vi "CameraSetParams.vi"(8 "error in (no error)":errorcluster, 10 "settings":T2={"exposure"=0.0, "external"=FALSE, "roi"={"left"=0, "top"=0, "right"=0, "bottom"=0}, "frames"=0, "binning"={"x"=1, "y"=1}}, 11 "NIvision in":refnum<class "IMAQdx.lvclass">) -> (0 "error out":errorcluster, 1 "roi_out":T1, 2 "attributes":variant[](array[variant]), 3 "NIvision out":refnum<class "IMAQdx.lvclass">)   [LabVIEW 2010, in "IMAQdx.lvclass"]
uses:
  <userlib>/bias/classes/IMAQdx/IMAQdx.lvclass
  <userlib>/bias/subvis/ExposureSettings.ctl
  <userlib>/bias/subvis/ROI_rect.ctl
  <vilib>/vision/driver/IMAQdx.llb/IMAQdx Acquisition Mode.ctl
  <userlib>/bias/classes/IMAQdx/IMAQdx.lvclass/IMAQdx.ctl
  <vilib>/vision/driver/NI_Vision_Acquisition_Software.lvlib
  resource/objmgr/imaqdx.rc
panel:
  out "ValueDBL":dbl
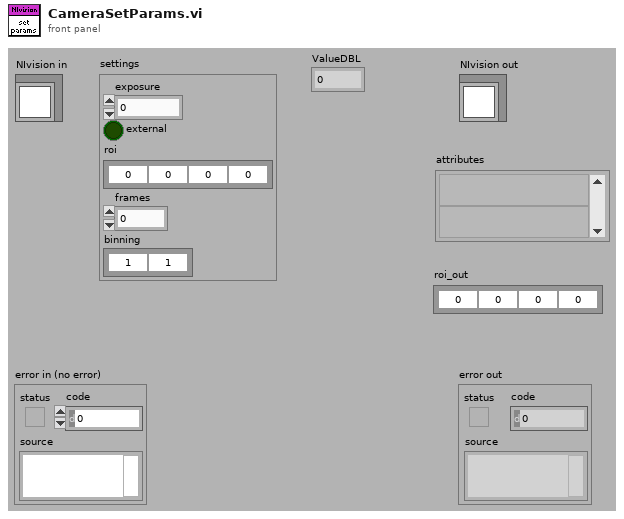
[diagram p1: front panel]
types:
  T1 = typedef "ROI_rect.ctl" = cluster{"left":i32, "top":i32, "right":i32, "bottom":i32}
  T2 = typedef "ExposureSettings.ctl" = cluster{"exposure":dbl, "external":bool, "roi":T1, "frames":i32, "binning":cluster{"x":u8, "y":u8}}
  T3 = typedef "NI_Vision_Acquisition_Software.lvlib/IMAQdx Acquisition Mode.ctl" = enum32{"One Shot", "Continuous"}
  T4 = typedef "IMAQdx.ctl" = refnum<k21>
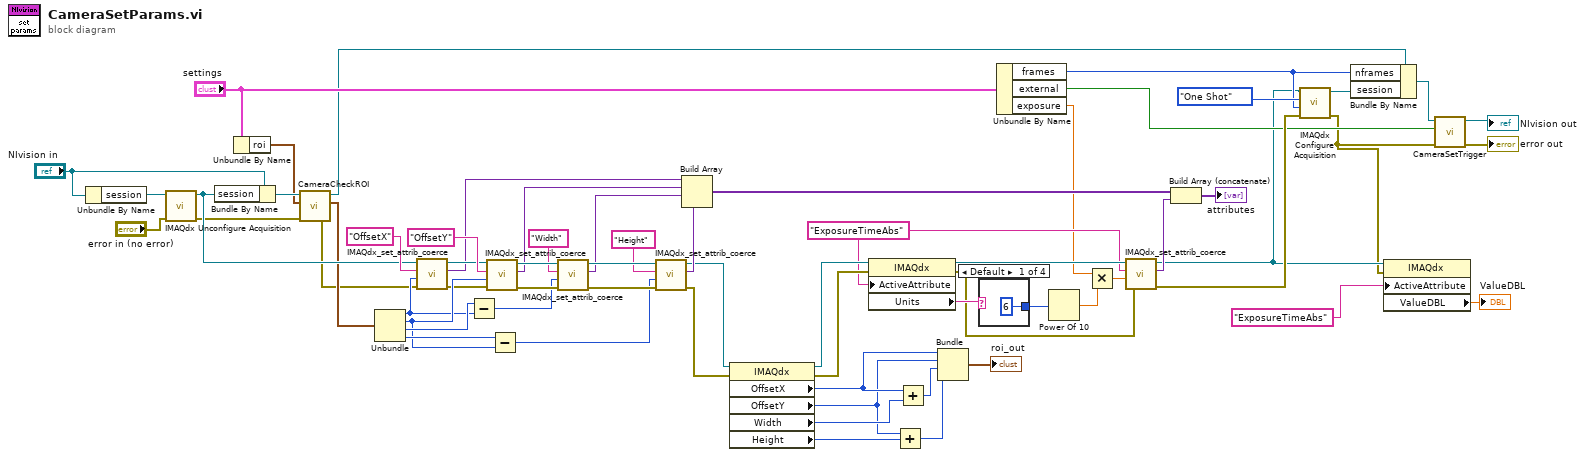
[diagram p0: block diagram]
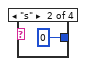
[diagram p2: hidden frame]
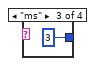
[diagram p3: hidden frame]
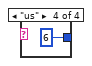
[diagram p4: hidden frame]
diagram:
  w29 = "ExposureTimeAbs" ("ActiveAttribute")
  n1 = Unbundle By Name("NIvision in") -> ("session"=w26:refnum<k21>)
  n2 = call <vilib>:"IMAQdx Unconfigure Acquisition.vi"("error in"="error in (no error)", "Session In"=w26) -> ("error out"=w11:errorcluster, "Session Out"=w17:T4)  [unwired: 8 in]
  n3 = Bundle By Name(cluster="NIvision in", "session"=w17) -> (w15:refnum<class "IMAQdx.lvclass">)
  n4 = Unbundle By Name("settings") -> ("roi"=w13:T1)
  n5 = call-dynamic "CameraCheckROI.vi"("error in (no error)"=w11, "ROI_in"=w13, "IMAQdx in"=w15) -> ("error out"=w10:errorcluster, "ROI_out"=w12:T1, "IMAQdx out"=w14:refnum<class "IMAQdx.lvclass">)  [unwired: 6 in]
  n6 = Unbundle(w12) -> ("left"=w55:i32, "top"=w59:i32, "right"=w65:i32, "bottom"=w62:i32)
  n7 = call <userlib>:"IMAQdx_set_attrib_coerce.vi"("error in"=w10, "value"=w55, "attribute"="OffsetX", "IMAQdx in"=w17) -> ("error out"=w58:errorcluster, "attrib out"=w56:variant, "IMAQdx out"=w57:T4)  [unwired: 1 out]
  n8 = Subtract(x=w65, y=w55) -> (x-y=w50:i32)
  n9 = call <userlib>:"IMAQdx_set_attrib_coerce.vi"("error in"=w58, "value"=w59, "attribute"="OffsetY", "IMAQdx in"=w57) -> ("error out"=w53:errorcluster, "attrib out"=w48:variant, "IMAQdx out"=w54:T4)  [unwired: 1 out]
  n10 = Subtract(x=w62, y=w59) -> (x-y=w49:i32)
  n11 = call <userlib>:"IMAQdx_set_attrib_coerce.vi"("error in"=w53, "value"=w50, "attribute"="Width", "IMAQdx in"=w54) -> ("error out"=w51:errorcluster, "attrib out"=w47:variant, "IMAQdx out"=w52:T4)  [unwired: 1 out]
  n12 = call <userlib>:"IMAQdx_set_attrib_coerce.vi"("error in"=w51, "value"=w49, "attribute"="Height", "IMAQdx in"=w52) -> ("error out"=w34:errorcluster, "attrib out"=w46:variant, "IMAQdx out"=w32:T4)  [unwired: 1 out]
  n13 = Build Array(w56, w48, w47, w46) -> (w43:variant[])
  n14 = property class="IMAQdx"(reference=w32, error in=w34) -> (reference out=w31:T4, error out=w33:errorcluster, "OffsetX"=w40:u32, "OffsetY"=w39:u32, "Width"=w41:u32, "Height"=w42:u32)
  n15 = property class="IMAQdx"(reference=w31, error in=w33, "ActiveAttribute"=w29) -> (reference out=w30:T4, error out=w28:errorcluster, "Units"=w63:string)
  n16 = Add(x=w39, y=w42) -> (x+y=w37:u32)
  n17 = Add(x=w40, y=w41) -> (x+y=w38:u32)
  n18 = Bundle("OffsetX"=w40, "OffsetY"=w39, w38, w37) -> (→"roi_out":cluster{"OffsetX":u32, "OffsetY":u32, u32, u32})  [unwired: 1 in]
  n19 = case shown="Default" w63 {
    tunnel: [6 ("y") 0 ("y") 3 ("y") 6 ("y")] -> w8
    frame Default {
    }
    frame "s" {
    }
    frame "ms" {
    }
    frame "us" {
    }
  }
  n20 = Unbundle By Name("settings") -> ("frames"=w19:i32, "external"=w16:bool, "exposure"=w5:dbl)
  n21 = Power Of 10(x=w8) -> (10^x=w7:dbl)
  n22 = Multiply(x=w5, y=w7) -> (x*y=w6:dbl)
  n23 = call <userlib>:"IMAQdx_set_attrib_coerce.vi"("error in"=w28, "value"=w6, "attribute"=w29, "IMAQdx in"=w30) -> ("error out"=w20:errorcluster, "attrib out"=w27:variant, "IMAQdx out"=w4:T4)  [unwired: 1 out]
  n24 = Build Array (concatenate)(w43, w27) -> (→"attributes":variant[])
  n25 = call <vilib>:"IMAQdx Configure Acquisition.vi"("error in"=w20, "Number of Buffers"=w19, "Continuous?"=IMAQdx_Acquisition_Mode."One Shot", "Session In"=w4) -> ("error out"=w3:errorcluster, "Session Out"=w22:T4)  [unwired: 6 in]
  n26 = Bundle By Name(cluster=w14, "nframes"=w19, "session"=w22) -> (w9:refnum<class "IMAQdx.lvclass">)
  n27 = property class="IMAQdx"(reference=w4, error in=w3, "ActiveAttribute"="ExposureTimeAbs") -> ("ValueDBL"=→"ValueDBL":dbl)  [unwired: 2 out]
  n28 = call-dynamic "CameraSetTrigger.vi"("error in (no error)"=w3, "external?"=w16, "IMAQdx in"=w9) -> ("error out"=→"error out":errorcluster, "IMAQdx out"=→"NIvision out":refnum<class "IMAQdx.lvclass">)  [unwired: 6 in, 1 out]
